vi "SafetyDataDisplay1.vi"(11 "data":bool[](array[boolean])) -> (3 "Table Control":string[][](table))   [LabVIEW 2026]
panel:
  in  "channel name":string[](array[string])=["14KS1", "14KS2", "Steering Position Reset", "Emergency Contactor", "IN SDA", "Battery Main ON Backup", "Low Battery", "Lexium Drive OK", "Rack & Pinion Steering Rack Present", "Electric Pump Test Bench Present", "Emergency Stop Status", "Lexium Drive Rack Braking OK", "Rack Extra Travel Right", "Rack Extra Track Left"]
  out "data":bool[](array[boolean])
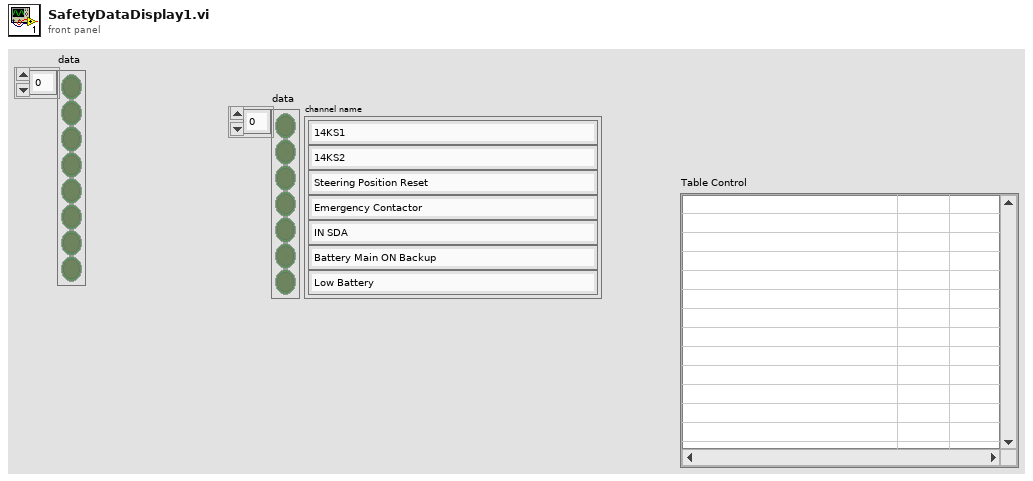
[diagram p1: front panel]
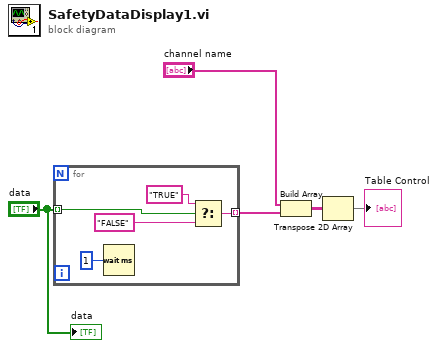
[diagram p0: block diagram]
diagram:
  n1 = for {
    tunnel: "data" -> [w9] mode=indexing
    tunnel: [w8] -> w2 mode=indexing
    n2 = Wait (ms)(milliseconds to wait=u32 1) -> ()  [unwired: 1 out]
    n3 = Select(t="TRUE", s=w9, f="FALSE") -> (s? t:f=w8:string)
  }
  n4 = Build Array("channel name", w2) -> (w4:string[][])
  n5 = Transpose 2D Array(2D array=w4) -> (transposed array=→"Table Control":string[][])
  "data" <- "data"
